vi "Binary Addition.vi"(10 "NUM 2 (Binary)":i32 format="%b", 11 "NUM 1 (Binary)":i32 format="%b") -> (3 "SUM (Binary)":i32 format="%b")   [LabVIEW 2020]
doc: "This VI will add two Binary Numbers."
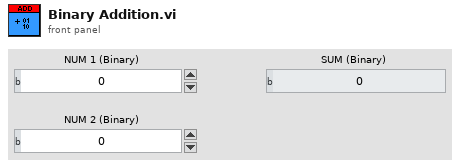
[diagram p1: front panel]
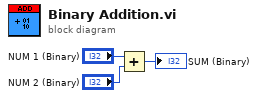
[diagram p0: block diagram]
diagram:
  n1 = Add(x="NUM 1 (Binary)", y="NUM 2 (Binary)") -> (x+y=→"SUM (Binary)":i32)
